vi "measure.vi"(0 "VISA resource name I":refnum<visa-resource-name>, 5 "Trigger Channel":i32(ring)=3 items=["Channel 1", "Channel 2", "Channel 3", "Channel 4", "External"], 7 "Testing?":bool, 9 "Channels":i32[](array[numeric]), 11 "error in":errorcluster) -> (4 "VISA resouce name O":refnum<visa-resource-name>, 6 "measurement results":waveform(dbl)[](array[waveform]), 10 "Tuning results":waveform(dbl)[](graph), 15 "error out":errorcluster)   [LabVIEW 2026]
uses:
  <instrlib>/Agilent 2000 3000 X-Series/Public/Data/Read Waveforms (Multiple).vi
  <instrlib>/Agilent 2000 3000 X-Series/Agilent 2000 3000 X-Series.lvlib
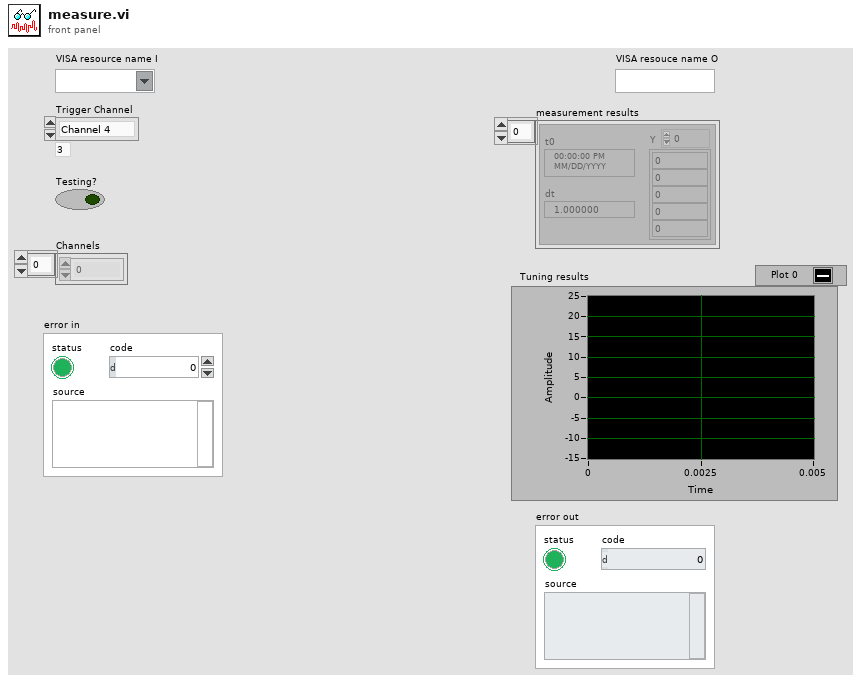
[diagram p1: front panel]
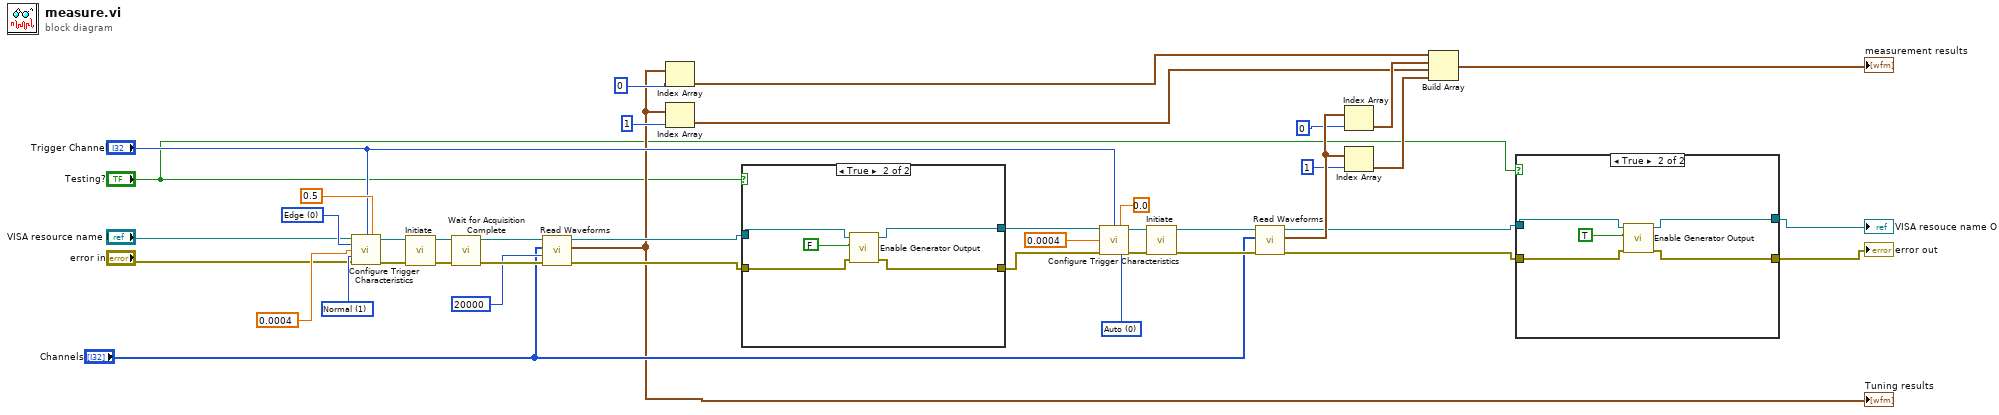
[diagram p0: block diagram]
diagram:
  w25 = 0 items=["Auto", "Normal"] ("Trigger Sweep (0: Auto)")
  w38 = 0 items=["Edge", "Glitch", "Pattern", "TV", "Edge Burst", "Runt", "Setup Hold", "Transition", "Serial Bus 1", "Serial Bus 2", "USB", "Delay", "Or", "Near Field Communication"] ("Trigger Type (0: Edge)")
  w40 = 1 items=["Auto", "Normal"] ("Trigger Sweep (0: Auto)")
  n1 = call <instrlib>:"Configure Trigger Characteristics.vi"("VISA resource name"="VISA resource name I", "Trigger Level Source (0: Channel 1)"="Trigger Channel", "Low Trigger Voltage Level (1 V)"=0.5, "Trigger Type (0: Edge)"=w38, "Holdoff Time (4E-8 S)"=0.0004, "Trigger Sweep (0: Auto)"=w40, "error in (no error)"="error in") -> ("VISA resource name out"=w42:refnum<visa-resource-name>, "error out"=w41:errorcluster)  [unwired: 7 in]
  n2 = call <instrlib>:"Initiate.vi"("error in (no error)"=w41, "VISA resource name"=w42) -> ("error out"=w28:errorcluster, "VISA resource name out"=w29:refnum<visa-resource-name>)  [unwired: 8 in]
  n3 = call <instrlib>:"Wait for Acquisition Complete.vi"("error in (no error)"=w28, "VISA resource name"=w29) -> ("error out"=w33:errorcluster, "VISA resource name out"=w34:refnum<visa-resource-name>)  [unwired: 8 in]
  n4 = call-poly <instrlib>:"Read Waveforms.vi"("error in (no error)"=w33, "Timeout (10000 ms)"=u32 20000, "Channels"="Channels", "VISA resource name"=w34) -> ("error out"=w19:errorcluster, "Waveform Data"=w6:waveform(dbl)[], "VISA resource name out"=w20:refnum<visa-resource-name>)  [unwired: 5 in]
  "Tuning results" <- w6
  n5 = Index Array(array=w6, index=0) -> (element=w11:waveform(dbl))
  n6 = Index Array(array=w6, index=1) -> (element=w9:waveform(dbl))
  n7 = case shown="True" "Testing?" {
    tunnel: w20 -> [w44 w49]
    tunnel: w19 -> [w43 w48]
    tunnel: [w44 w47] -> w22
    tunnel: [w43 w46] -> w21
    frame False {
    }
    frame True {
      n8 = call <instrlib>:"Enable Generator Output.vi"("error in (no error)"=w48, "Enable Output (F: Disable)"=FALSE, "VISA resource name"=w49) -> ("error out"=w46:errorcluster, "VISA resource name out"=w47:refnum<visa-resource-name>)  [unwired: 7 in]
    }
  }
  n9 = call <instrlib>:"Configure Trigger Characteristics.vi"("VISA resource name"=w22, "Trigger Level Source (0: Channel 1)"="Trigger Channel", "Low Trigger Voltage Level (1 V)"=0.0, "Holdoff Time (4E-8 S)"=0.0004, "Trigger Sweep (0: Auto)"=w25, "error in (no error)"=w21) -> ("VISA resource name out"=w27:refnum<visa-resource-name>, "error out"=w26:errorcluster)  [unwired: 8 in]
  n10 = call <instrlib>:"Initiate.vi"("error in (no error)"=w26, "VISA resource name"=w27) -> ("error out"=w13:errorcluster, "VISA resource name out"=w14:refnum<visa-resource-name>)  [unwired: 8 in]
  n11 = call-poly <instrlib>:"Read Waveforms.vi"("error in (no error)"=w13, "Channels"="Channels", "VISA resource name"=w14) -> ("error out"=w4:errorcluster, "Waveform Data"=w17:waveform(dbl)[], "VISA resource name out"=w5:refnum<visa-resource-name>)  [unwired: 6 in]
  n12 = Index Array(array=w17, index=0) -> (element=w10:waveform(dbl))
  n13 = Index Array(array=w17, index=1) -> (element=w8:waveform(dbl))
  n14 = Build Array(w11, w10, w9, w8) -> (→"measurement results":waveform(dbl)[])
  n15 = case shown="True" "Testing?" {
    tunnel: w5 -> [w51 w56]
    tunnel: w4 -> [w50 w55]
    tunnel: [w51 w54] -> w2
    tunnel: [w50 w53] -> w1
    frame False {
    }
    frame True {
      n16 = call <instrlib>:"Enable Generator Output.vi"("error in (no error)"=w55, "Enable Output (F: Disable)"=TRUE, "VISA resource name"=w56) -> ("error out"=w53:errorcluster, "VISA resource name out"=w54:refnum<visa-resource-name>)  [unwired: 7 in]
    }
  }
  "VISA resouce name O" <- w2
  "error out" <- w1
